vi "Method Tuner.vi"(0 "Method File:":path=path "C:/Users/Min/Documents/Software Design/Requests/Method Tunner/Mode Switching-ESI1-APCI2-Molana.xml") -> ()   [LabVIEW 2012]
uses:
  _XML Source Type.ctl
  _Source Parameter.ctl
  <vilib>/xml/Close Reference(Node).vi
  <vilib>/xml/NI_XML.lvlib
  <resource>/objmgr/DOMUserDefRef.rc
panel:
  out "xml":string
  in  "Load":bool
  in  "Save":bool
  in  "Current Expt":u16(ring) items=["0", "1"]
  in  "Tab":T1(tab)=enum."Experiments"
  out "Method-Level Parameter":string[][](table)
  out "Experiment List":string[][](table)
  out "Expt Comment":string
  out "Expt-Level Parameter":string[][](table)
  out "Source Type":T2 items=["APCI 1", "APCI 2", "ESI 1", "ESI 2"]
  out "Expt-Level Source Parameters":T3
  out "Mass Ranges":string[][](table)
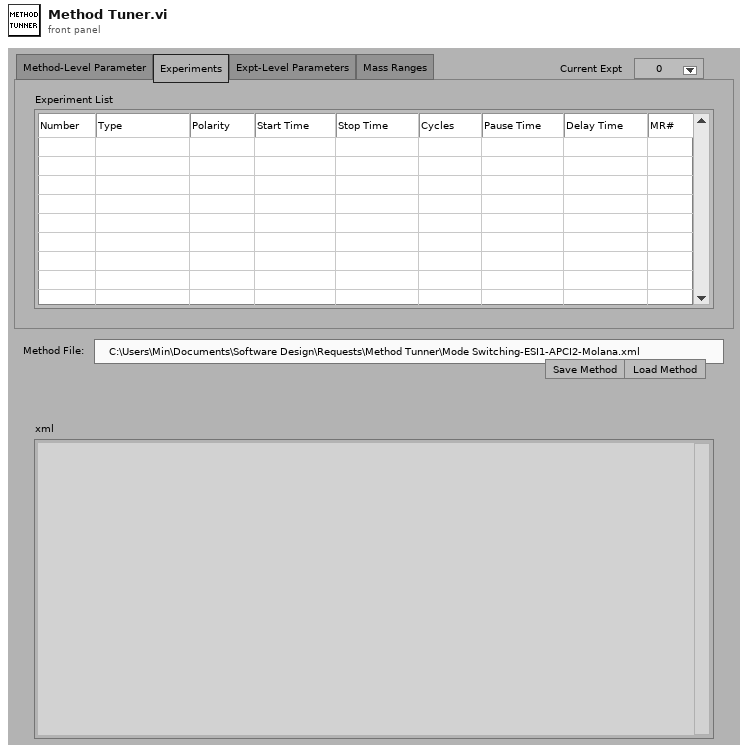
[diagram p1: front panel]
types:
  T1 = enum32{"Method-Level Parameter", "Experiments", "Expt-Level Parameters", "Mass Ranges"}
  T2 = typedef "_XML Source Type.ctl" = u16
  T3 = typedef "_Source Parameter.ctl" = cluster{"Corona Discharge: ":dbl, "ElectroSpray V1: ":dbl, "ElectroSpray V2: ":dbl}
  T4 = enum32{"existing file", "new file", "new or existing file", "existing dir", "new dir", "new or existing dir", "existing file (use LLBs)", "new file (use LLBs)", "new or existing file (use LLBs)", "new or existing file or directory (use LLBs)"}
  T5 = typedef "_Mass Range Parameters.ctl" = cluster{"Name":string, "Ch#":u8, "StartV":dbl, "StopV":dbl, "StepV":dbl, "Index":u8}
  T6 = cluster{"ExptLevelParameters":string[][], "MassRanges":string[][], " MRParameters":T5[][]}
  T7 = cluster{"ExptLevelParameters":string[][], "MassRanges":string[][], " MRParameters":T5[][]}[]
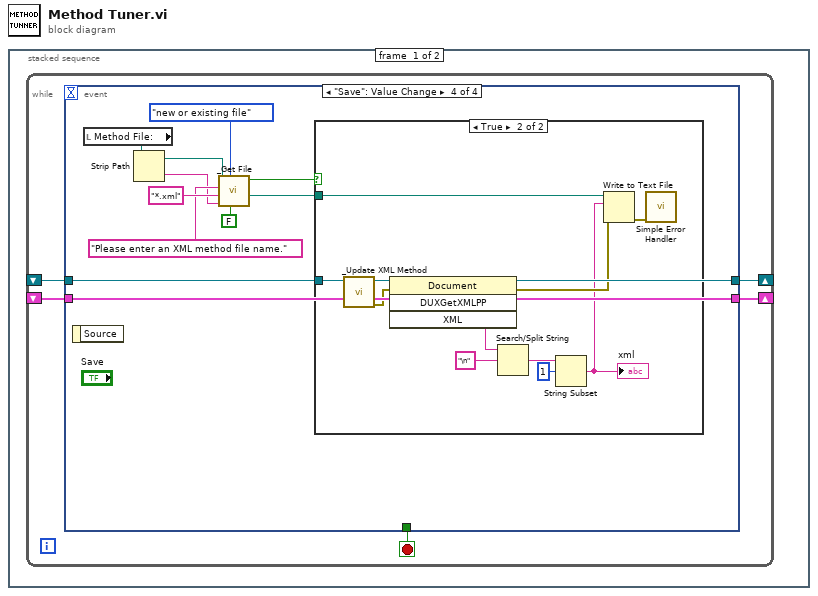
[diagram p0: block diagram]
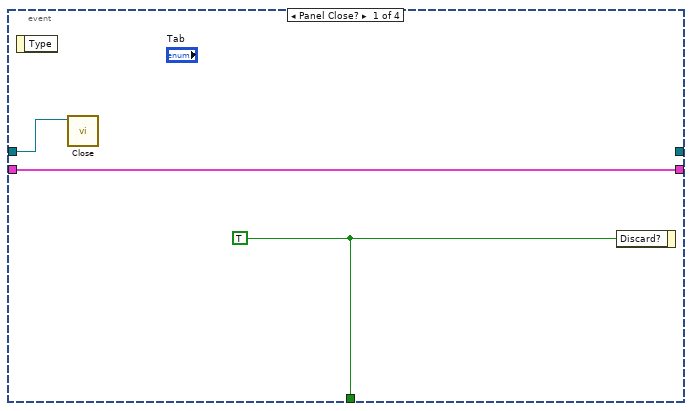
[diagram p2: hidden frame]
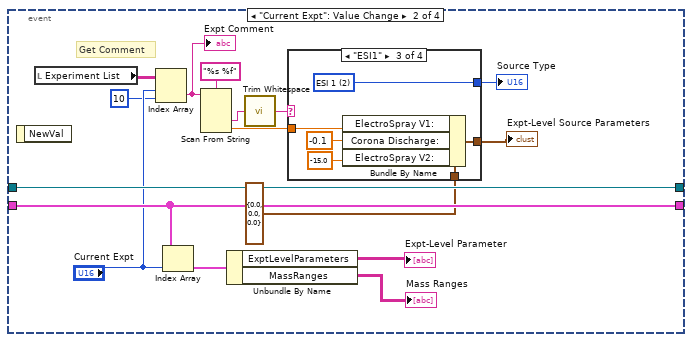
[diagram p3: hidden frame]
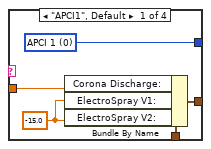
[diagram p4: hidden frame]
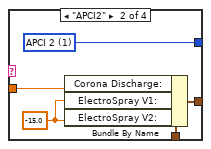
[diagram p5: hidden frame]
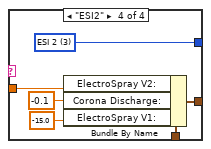
[diagram p6: hidden frame]
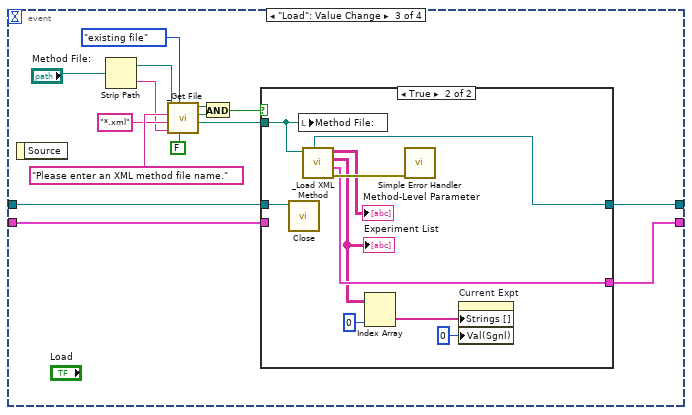
[diagram p7: hidden frame]
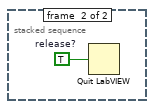
[diagram p10: hidden frame]
diagram:
  n1 = stacked-sequence {
    frame #0 {
      n2 = while {
        shift-right: [w3] -> _
        shift-left: _ -> [w4]
        shift-right: [w1] -> _
        shift-left: _ -> [w2]
        stop <- w5 stop-if-true
        n3 = event shown="[3] \"Save\": Value Change" {
          selector: _ -> [_ _ _ _]
          dyn-events: _ -> [_ _ _ _]
          timeout: _ -> [_ _ _ _]
          tunnel: [w8 _ _ _] -> w5
          tunnel: w4 -> [w7 w24 w52 w74]
          tunnel: [w7 w24 w53 w74] -> w3
          tunnel: w2 -> [w6 w20 w51 w75]
          tunnel: [_ w20 w50 w75] -> w1
          event Panel Close? {
            w8 = TRUE ("Discard?")
            n4 = event-data() -> ()  [unwired: 2 out]
            n5 = call-poly <vilib>:"Close.vi"("node"=w6) -> ()  [unwired: 8 in, 1 out]
            n6 = event-data("Discard?"=w8) -> ()  [unwired: 1 in, 1 out]
          }
          event "Current Expt": Value Change {
            # "Get Comment"
            n7 = event-data() -> ()  [unwired: 2 out]
            n8 = local read "Experiment List"() -> (w19:string[][])
            n9 = Index Array(array=w19, index (row)="Current Expt", index (col)=10 ("disabled index (col)")) -> (element=w15:string)
            "Expt Comment" <- w15
            n10 = Index Array(array=w24, index="Current Expt") -> (element=w23:T6)
            n11 = Scan From String(format string="%s %f", input string=w15) -> (output 1=w14:string, output 2=w10:dbl)  [unwired: 4 in, 3 out]
            n12 = Unbundle By Name(w23) -> ("ExptLevelParameters"=→"Expt-Level Parameter":string[][], "MassRanges"=→"Mass Ranges":string[][])
            n13 = call <vilib>:"Trim Whitespace.vi"("string"=w14) -> ("trimmed string"=w13:string)  [unwired: 1 in]
            n14 = case shown="\"ESI1\"" w13 {
              tunnel: [w29 w34 w40 w46] -> w12
              tunnel: T3 {"Corona Discharge: "=0.0, "ElectroSpray V1: "=0.0, "ElectroSpray V2: "=0.0} ("Method-Level Source Parameters") -> [w28 w32 w37 w45]
              tunnel: w10 -> [w27 w31 w36 w44]
              tunnel: [w25 w30 w35 w41] -> w9
              frame "APCI1", Default {
                w26 = -15.0 ("ElectroSpray V2:")
                w29 = T2 0 items=["APCI 1", "APCI 2", "ESI 1", "ESI 2"] ("Source Type")
                n15 = Bundle By Name(cluster=w28, "Corona Discharge:"=w27, "ElectroSpray V1:"=w26, "ElectroSpray V2:"=w26) -> (w25:T3)
              }
              frame "APCI2" {
                w33 = -15.0 ("ElectroSpray V2:")
                w34 = T2 1 items=["APCI 1", "APCI 2", "ESI 1", "ESI 2"] ("Source Type")
                n16 = Bundle By Name(cluster=w32, "Corona Discharge:"=w31, "ElectroSpray V1:"=w33, "ElectroSpray V2:"=w33) -> (w30:T3)
              }
              frame "ESI1" {
                w40 = T2 2 items=["APCI 1", "APCI 2", "ESI 1", "ESI 2"] ("Source Type")
                n17 = Bundle By Name(cluster=w37, "ElectroSpray V1:"=w36, "Corona Discharge:"=-0.1, "ElectroSpray V2:"=-15.0) -> (w35:T3)
              }
              frame "ESI2" {
                w46 = T2 3 items=["APCI 1", "APCI 2", "ESI 1", "ESI 2"] ("Source Type")
                n18 = Bundle By Name(cluster=w45, "ElectroSpray V2:"=w44, "Corona Discharge:"=-0.1, "ElectroSpray V1:"=-15.0 ("ElectroSpray V2:")) -> (w41:T3)
              }
            }
            "Source Type" <- w12
            "Expt-Level Source Parameters" <- w9
          }
          event "Load": Value Change {
            n19 = event-data() -> ()  [unwired: 2 out]
            n20 = Strip Path(path="Method File:") -> (stripped path=w48:path, name=w47:string)
            n21 = call "_Get File.vi"("For Write (T)"=FALSE, "select mode (new or existing)"=T4."existing file", "default name"=w47, "extension (isd)"="*.xml", "prompt"="Please enter an XML method file name.", "Start Path"=w48) -> ("Seleted File"=w54:path, "Exists"=w56:bool, "Succeeded"=w57:bool)  [unwired: 1 in]
            n22 = And(x=w57, y=w56) -> (x .and. y?=w55:bool)
            n23 = case shown="True" w55 {
              tunnel: w54 -> [_ w73]
              tunnel: [w63 w70] -> w53
              tunnel: w52 -> [w63 _]
              tunnel: w51 -> [w62 w64]
              tunnel: [w62 w65] -> w50
              frame False {
              }
              frame True {
                n24 = call-poly <vilib>:"Close.vi"("node"=w64) -> ()  [unwired: 8 in, 1 out]
                n25 = local write "Method File:"(w73) -> ()
                n26 = call "_Load XML Method.vi"("Path"=w73) -> ("error out"=w72:errorcluster, "ExptParamAndMR"=w70:T7, "Experiment List"=w69:string[][], "MethodLevelParameters"=→"Method-Level Parameter":string[][], "DOM document"=w65:refnum<k20>)  [unwired: 3 in]
                "Experiment List" <- w69
                n27 = Index Array(array=w69, index (col)=0 ("disabled index (col)")) -> (element=w67:string[])  [unwired: 1 in]
                n28 = call <vilib>:"Simple Error Handler.vi"("error in (no error)"=w72) -> ()  [unwired: 4 in, 5 out]
                n29 = property on="Current Expt" class="Ring (strict)"("Strings []"=w67, "Val(Sgnl)"=u16 0 ("Value (Signaling)")) -> ()  [unwired: 2 in, 2 out]
              }
            }
          }
          event "Save": Value Change {
            n30 = event-data() -> ()  [unwired: 2 out]
            n31 = local read "Method File:"() -> (w80:path)
            n32 = Strip Path(path=w80) -> (stripped path=w79:path, name=w78:string)
            n33 = call "_Get File.vi"("For Write (T)"=FALSE, "select mode (new or existing)"=T4."new or existing file", "default name"=w78, "extension (isd)"="*.xml", "prompt"="Please enter an XML method file name.", "Start Path"=w79) -> ("Seleted File"=w76:path, "Succeeded"=w77:bool)  [unwired: 1 in, 1 out]
            n34 = case shown="True" w77 {
              tunnel: w76 -> [_ w93]
              tunnel: w75 -> [_ w95]
              frame False {
              }
              frame True {
                n35 = call "_Update XML Method.vi"("DOM document"=w95) -> ("error out"=w91:errorcluster, "DOM document out"=w94:refnum<k20>)  [unwired: 6 in]
                n36 = invoke class="Document" method="DUXGetXMLPP"(reference=w94, error in=w91) -> (error out=w90:errorcluster, "XML"=w89:string)  [unwired: 2 in, 2 out]
                n37 = Search/Split String(string=w89, search string/char (-)="\n") -> (match + rest of string=w86:string)  [unwired: 1 in, 2 out]
                n38 = String Subset(string=w86, offset (0)=1) -> (substring=w87:string)  [unwired: 1 in]
                "xml" <- w87
                n39 = Write to Text File(file (use dialog)=w93, text=w87, error in=w90) -> (error out=w92:errorcluster)  [unwired: 1 in, 2 out]
                n40 = call <vilib>:"Simple Error Handler.vi"("error in (no error)"=w92) -> ()  [unwired: 4 in, 5 out]
              }
            }
          }
        }
      }
    }
    frame #1 {
      w96 = TRUE  # release?
      n41 = Quit LabVIEW(quit? (T)=w96) -> ()
    }
  }
